vi "Events.vi"() -> ()   [LabVIEW 2022 SP3]
panel:
  in  "stop":bool
  in  "LED OF":bool
  out "Boolean":bool
  in  "LED ON":bool
  in  "String":string
  out "Numeric 2":dbl
  in  "Numeric":dbl
  in  "Slide":dbl(slide) scale=0.0..10.0
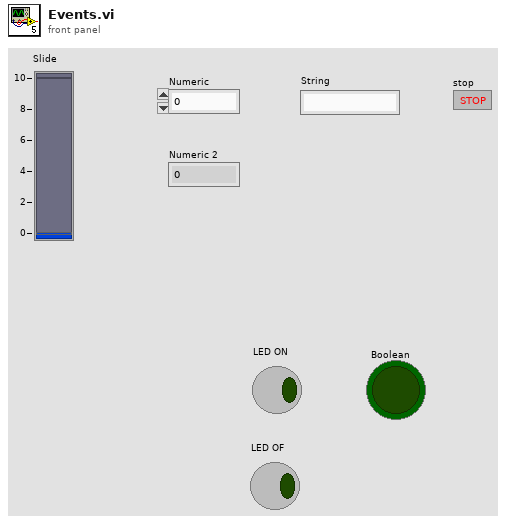
[diagram p1: front panel]
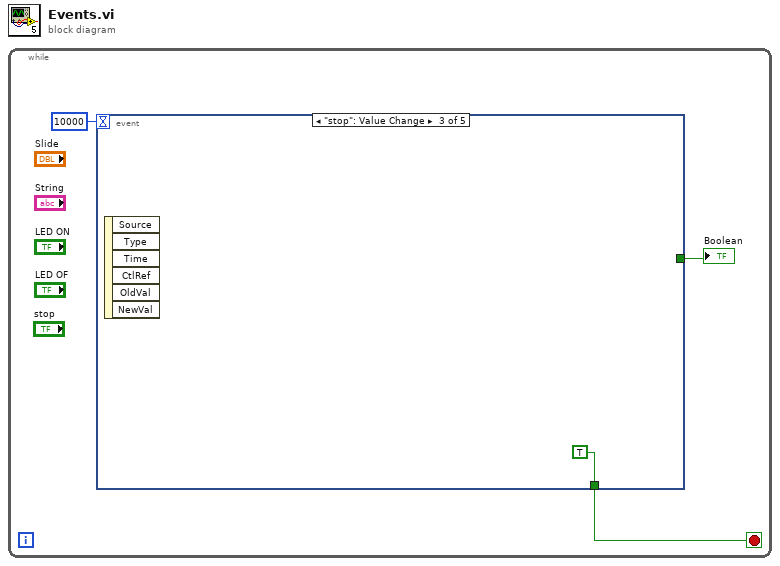
[diagram p0: block diagram]
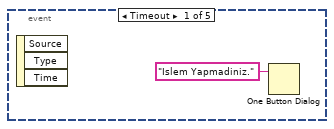
[diagram p2: hidden frame]
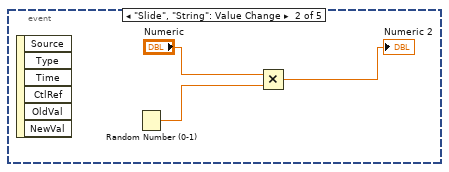
[diagram p3: hidden frame]
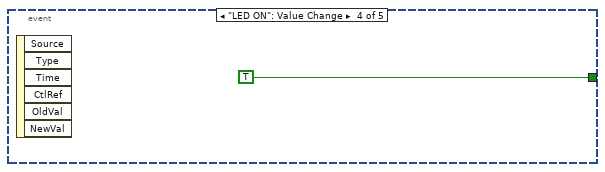
[diagram p4: hidden frame]
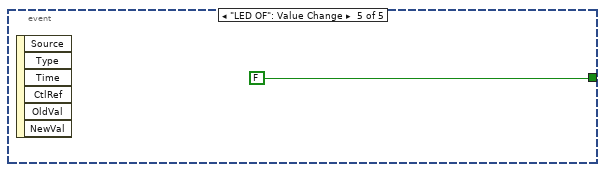
[diagram p5: hidden frame]
diagram:
  n1 = while {
    stop <- w1 stop-if-true
    n2 = event shown="[2] \"stop\": Value Change" {
      selector: _ -> [_ _ _ _ _]
      dyn-events: _ -> [_ _ _ _ _]
      timeout: 10000 -> [_ _ _ _ _]
      tunnel: [_ _ _ TRUE FALSE] -> w2
      tunnel: [_ _ TRUE _ _] -> w1
      event Timeout {
        n3 = event-data() -> ()  [unwired: 1 in, 3 out]
        n4 = One Button Dialog(message="Islem Yapmadiniz.") -> ()  [unwired: 1 in, 1 out]
      }
      event "Slide", "String": Value Change {
        n5 = event-data() -> ()  [unwired: 1 in, 6 out]
        n6 = Random Number (0-1)() -> (number: 0 to 1=w6:dbl)
        n7 = Multiply(x="Numeric", y=w6) -> (x*y=→"Numeric 2":dbl)
      }
      event "stop": Value Change {
        n8 = event-data() -> ()  [unwired: 1 in, 6 out]
      }
      event "LED ON": Value Change {
        n9 = event-data() -> ()  [unwired: 1 in, 6 out]
      }
      event "LED OF": Value Change {
        n10 = event-data() -> ()  [unwired: 1 in, 6 out]
      }
    }
    "Boolean" <- w2
  }
